vi "CPP_SpectraFit.vi"() -> (5 "Plug in titles":string[](array[string]), 7 "Plug in values":string[](array[string]))   [LabVIEW 2011]
uses:
  Controls/Instrument_Array.ctl
  Controls/Post_Process.ctl
  Controls/Graph_Type.ctl
  Globals/Meas_global.vi
panel:
  in  "Divider":i32(slide)=10 scale=1.0..100000.0 scale format="%#_6e"
  out "dF/ Hz":dbl
  in  "Show Smooth":bool=TRUE
  in  "Save Spectra?":bool
  in  "Desired number of samples per block":i32=32768
  out "Spectra":cluster{"Frequencies":dbl[], dbl[]}[](graph)
  in  "Averaging samples":i32=1 min=1 max=1000
  in  "Spectra Index (from ALL channels)":i32
  out "Waveform Graph":dbl[][](graph)
  in  "Channels to Plot":i32[](array[ring])=[0] items=["RV (Uref)", "Save Nothing"]
  # "Run this VI to update the channel names"
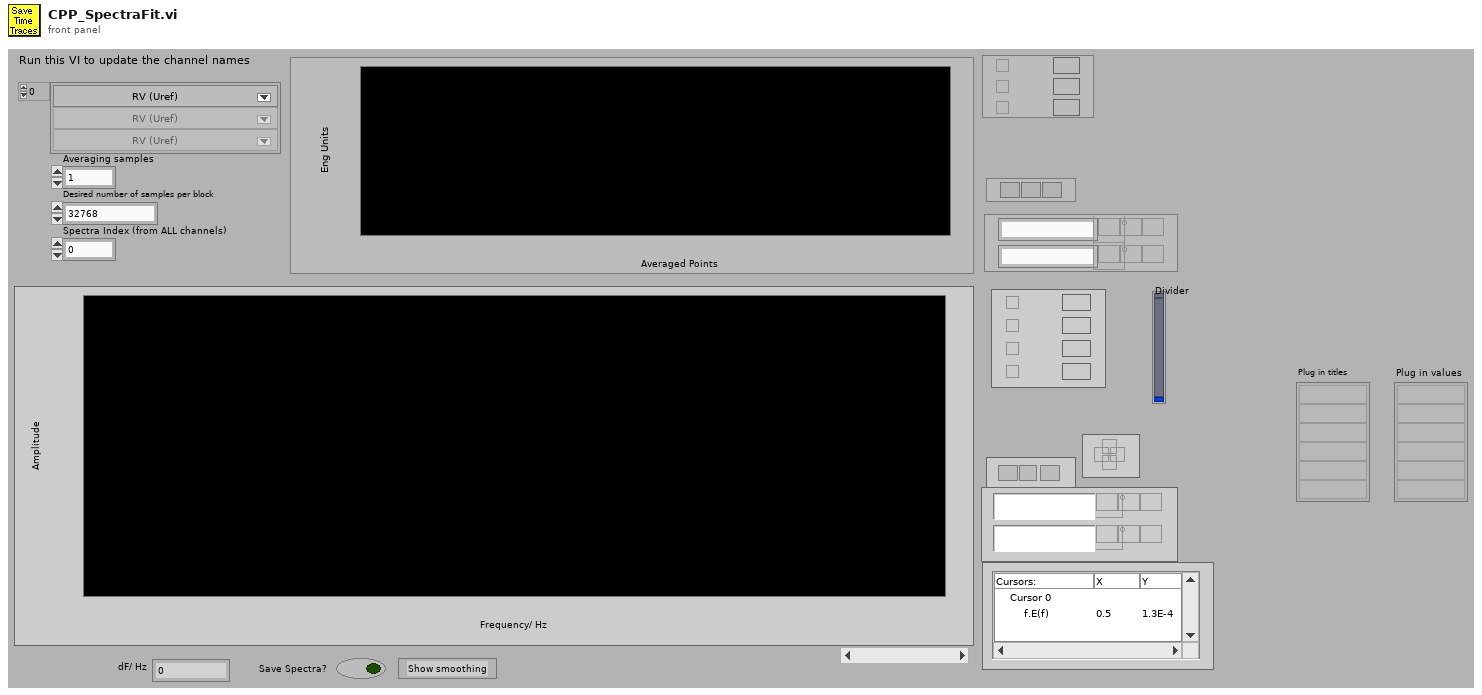
[diagram p1: front panel]
types:
  T1 = typedef "Analysis_info_cluster.ctl" = cluster{"Colour":u32, "Inst type":T2, "Inst name":string, "Symbol":string, "Code name":string, "Extra Info":string, "Inst Array":T3, "Extra Titles":string[], "Extra Values":string[], "U":dbl, "u^2":dbl, "u^3":dbl, "u^4":dbl, "Skew_u":dbl, "Kurt_u":dbl, "Sd Error in Mean":dbl, "% u'/U":dbl, "X":dbl, "Y":dbl, "Z":dbl, "Timescale integral to 25%":dbl, "Sd Error in Variance":dbl, "Calib File":path, "Calib Constants":dbl[], "Output Position":bool, "Full Stats":bool, "Av Sampling Rate":dbl, "Av No of Samples":dbl, "Total Meas Time (s)":dbl, "ADAM Ch Name":string}
  T2 = typedef "Inst_type.ctl" = enum16{"Propeller anemometer", "Raw voltage", "Pressure Transducer", "Pitot-static tube", "Preston tube", "Hot wire", "Cross wire 1", "Cross wire 2", "Generic Linear", "Generic Polynomial", "Generic BackPoly", "Fast FID", "Thermocouple", "Cold wire", "Pulsed Wire", "LDA Vel", "LDA Tran time", "LDA Arr time"}
  T3 = typedef "Instrument_Array.ctl" = enum16{"PWA", "LDA", "Analogue"}
  T4 = typedef "Post_Process.ctl" = enum16{"Take New Data", "Post Process Raw Data File"}
  T5 = typedef "Graph_Type.ctl" = enum16{"Show no graph", "Voltage trace", "Velocity trace", "Vel histogram", "Spectrum", "f.E(f) v Log f", "Auto-Corr"}
  T6 = cluster{"Plot 1":u16, "Plot 2":u16, "Save graph":u16, "Plot Type":T5}
  T7 = cluster{"Weighting":dbl[], "Time (ms)":dbl[], "Voltage":dbl[], "Eng Values":dbl[]}[]
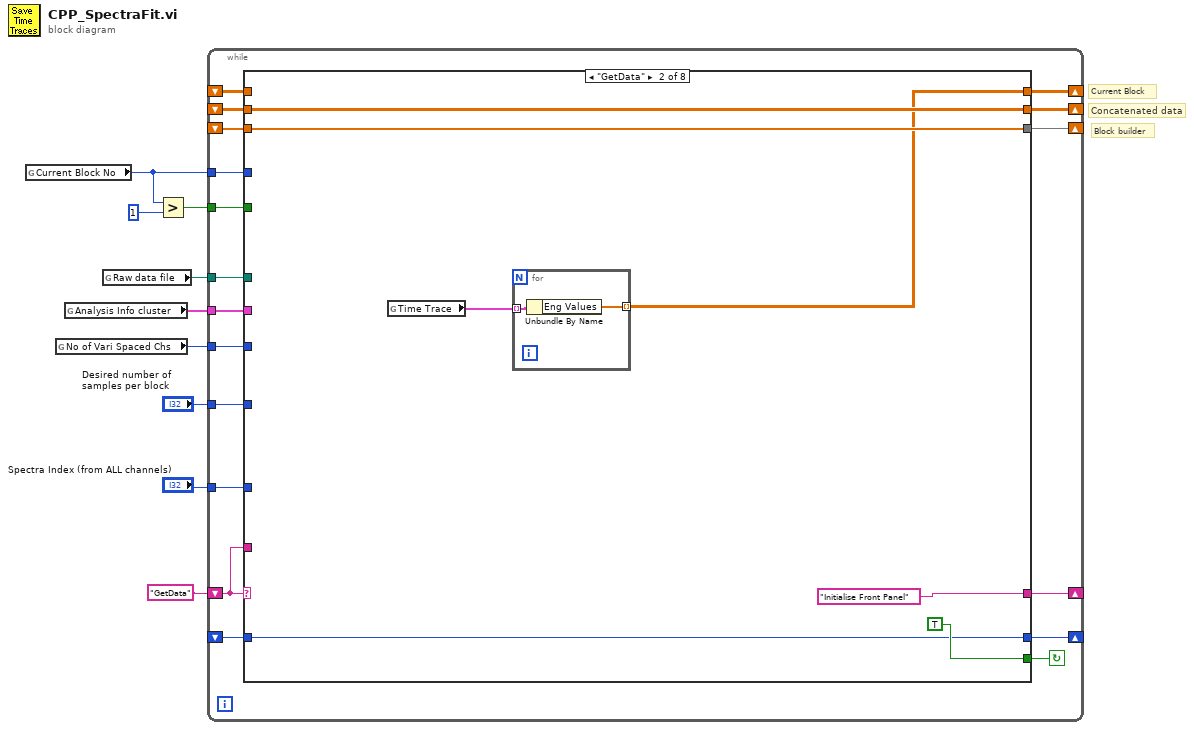
[diagram p0: block diagram]
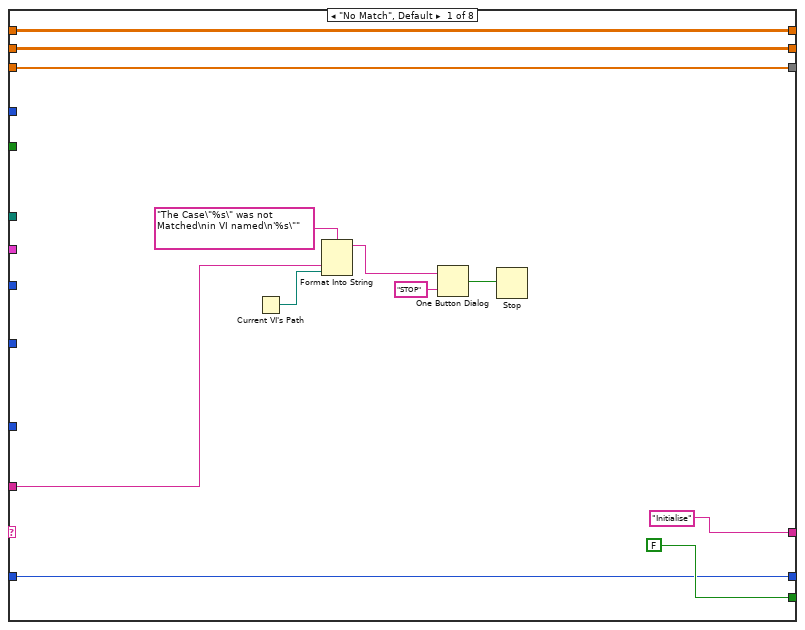
[diagram p2: hidden frame]
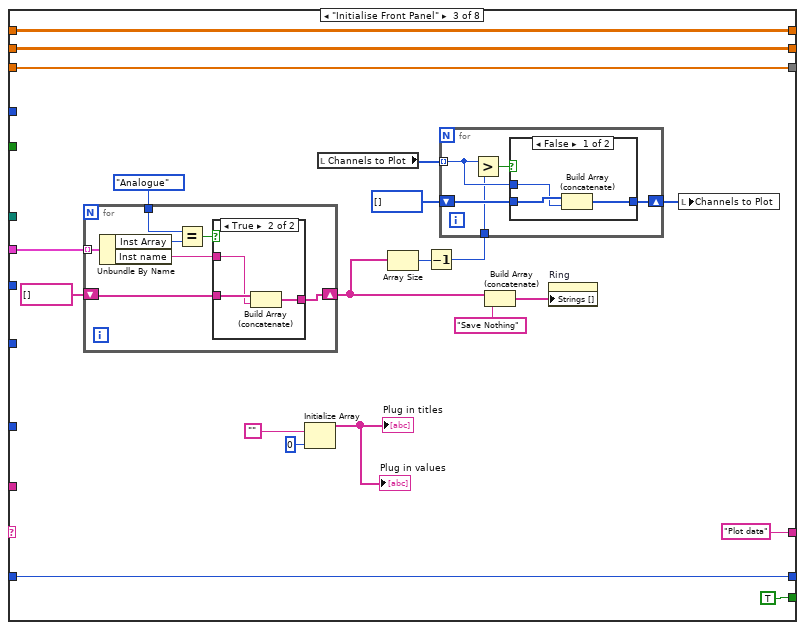
[diagram p3: hidden frame]
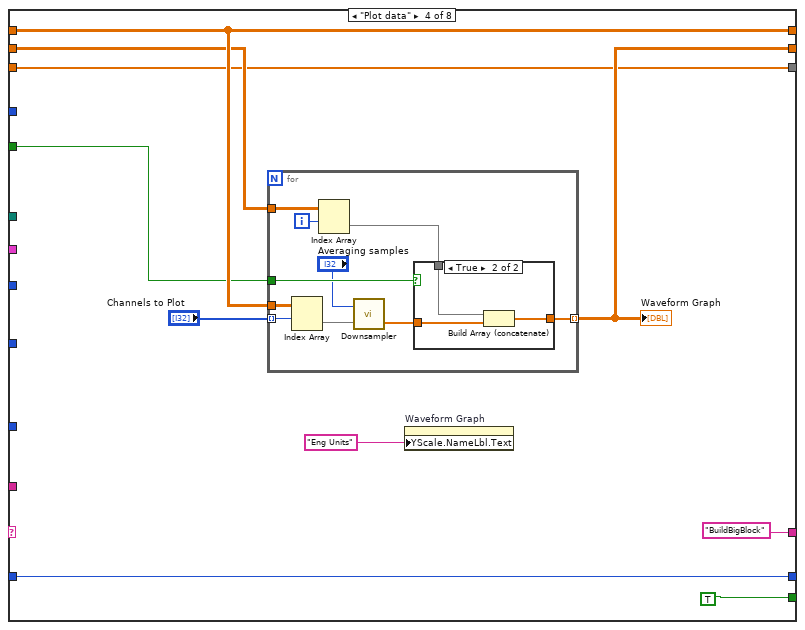
[diagram p6: hidden frame]
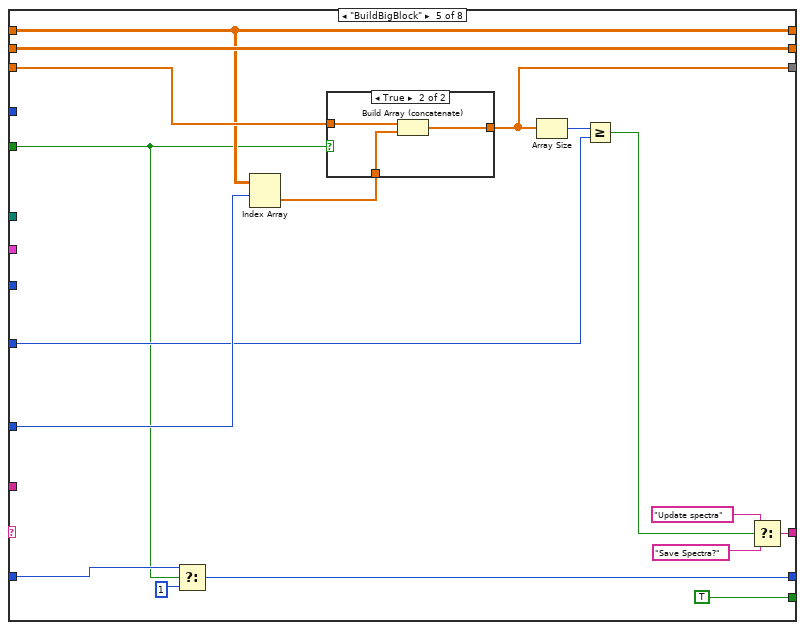
[diagram p8: hidden frame]
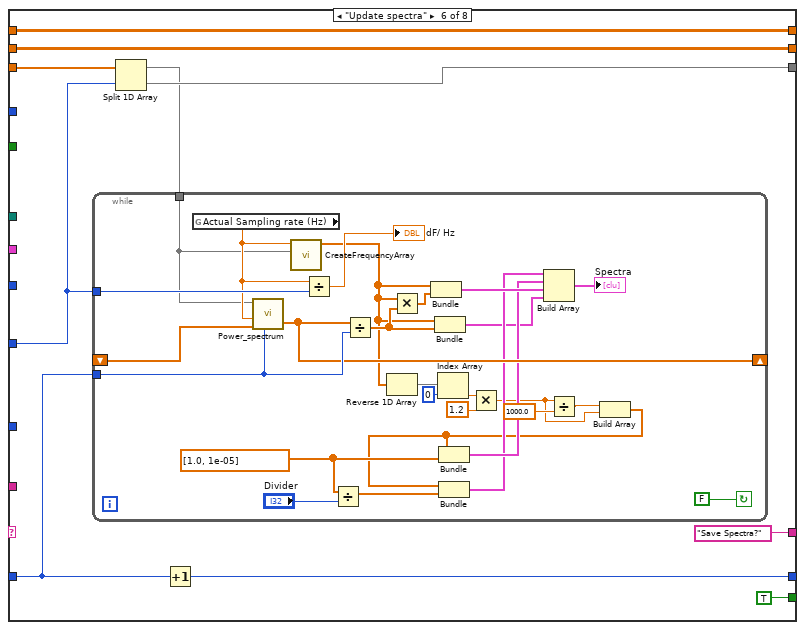
[diagram p10: hidden frame]
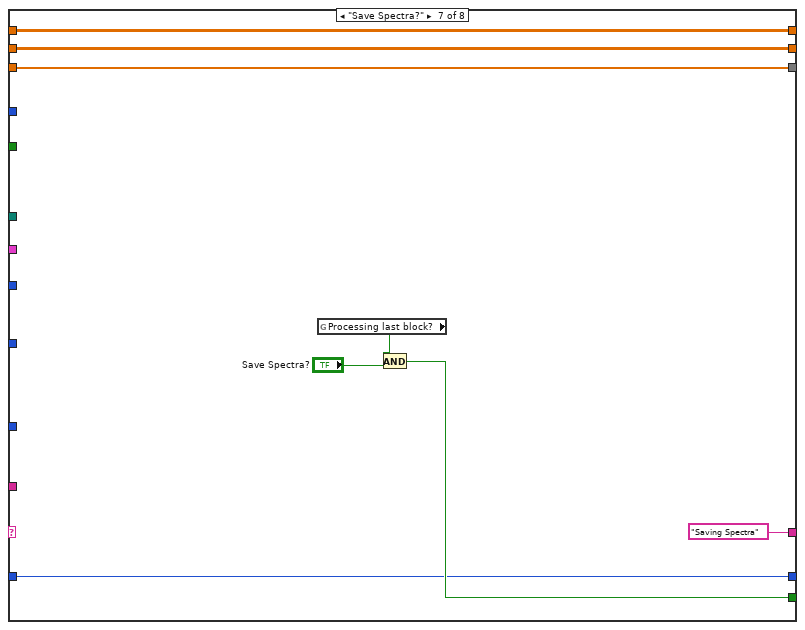
[diagram p11: hidden frame]
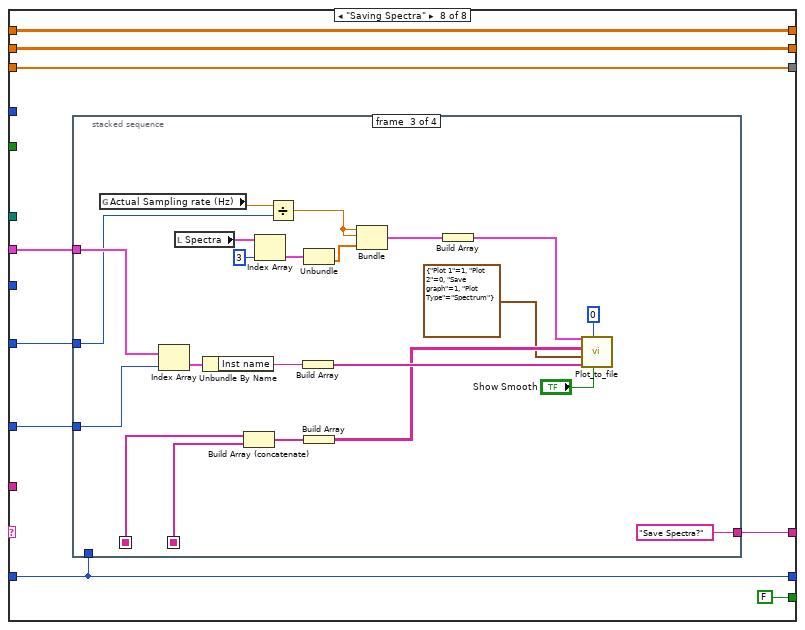
[diagram p12: hidden frame]
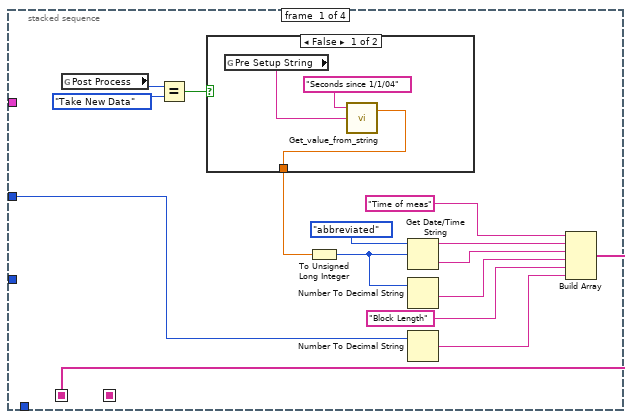
[diagram p13: hidden frame]
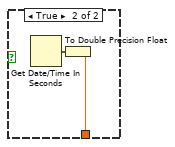
[diagram p14: hidden frame]
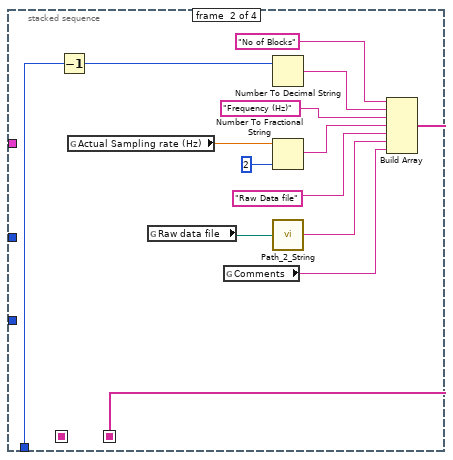
[diagram p15: hidden frame]
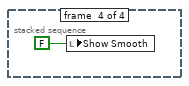
[diagram p16: hidden frame]
diagram:
  # "Block builder"
  # "Concatenated data"
  # "Current Block"
  n1 = global read "Meas_global.vi" "Current Block No"() -> (w6:i32)
  n2 = global read "Meas_global.vi" "No of Vari Spaced Chs"() -> (w4:i32)
  n3 = global read "Meas_global.vi" "Analysis Info cluster"() -> (w5:T1[])
  n4 = global read "Meas_global.vi" "Raw data file"() -> (w8:path)
  n5 = Greater?(x=w6, y=1) -> (0:w3:bool)
  n6 = while {
    shift-left: "GetData" -> [w25]
    shift-right: [w26] -> _
    tunnel: w8 -> [w24]
    tunnel: w3 -> [w23]
    tunnel: w6 -> [w22]
    tunnel: w5 -> [w21]
    tunnel: w4 -> [w20]
    shift-right: [w19] -> _
    shift-left: _ -> [w18]
    shift-right: [w16] -> _
    shift-left: _ -> [w17]
    shift-right: [w14] -> _
    shift-left: _ -> [w15]
    tunnel: "Desired number of samples per block" -> [w13]
    tunnel: "Spectra Index (from ALL channels)" -> [w12]
    shift-right: [w11] -> _
    shift-left: _ -> [w10]
    stop <- w27 continue-if-true
    n7 = case shown="\"GetData\"" w25 {
      tunnel: [FALSE TRUE TRUE TRUE ("Calculate Spectra and Histogram?") TRUE ("Calculate Spectra and Histogram?") TRUE ("Calculate Spectra and Histogram?") w172 FALSE ("Calculate Spectra and Histogram?")] -> w27
      tunnel: ["Initialise" "Initialise Front Panel" "Plot data" "BuildBigBlock" ("t") w114 "Save Spectra?" "Saving Spectra" w185] -> w26
      tunnel: w25 -> [w34 _ _ _ _ _ _ _]
      tunnel: w24 -> [_ _ _ _ _ _ _ _]
      tunnel: w23 -> [_ _ _ w96 w117 _ _ _]
      tunnel: w22 -> [_ _ _ _ _ _ _ _]
      tunnel: w21 -> [_ _ w52 _ _ _ _ w183]
      tunnel: w20 -> [_ _ _ _ _ _ _ _]
      tunnel: [w31 w40 w58 w98 w127 w142 w177 w186] -> w19
      tunnel: w18 -> [w31 _ w58 w98 w127 w142 w177 w186]
      tunnel: w17 -> [w30 w44 w57 w97 w128 w143 w178 w187]
      tunnel: [w30 w44 w57 w94 w128 w143 w178 w187] -> w16
      tunnel: w15 -> [w29 w43 w54 w92 w129 w141 w175 w184]
      tunnel: [w29 w43 w54 w92 w125 w140 w175 w184] -> w14
      tunnel: w13 -> [_ _ _ _ w121 w136 _ w180]
      tunnel: w12 -> [_ _ _ _ w123 _ _ w182]
      tunnel: [w28 w42 w53 w91 w118 w134 w171 w179] -> w11
      tunnel: w10 -> [w28 w42 w53 w91 w119 w135 w171 w179]
      frame "No Match", Default {
        n8 = Current VI's Path() -> (path=w33:path)
        n9 = Format Into String(format string="The Case\"%s\" was not Matched\nin VI named\n'%s\"" ("Format String"), w34, w33) -> (resulting string=w37:string)  [unwired: 2 in, 1 out]
        n10 = One Button Dialog(message=w37, button name ("OK")="STOP") -> (true=w35:bool)
        n11 = Stop(stop? (T)=w35) -> ()
      }
      frame "GetData" {
        n12 = global read "Meas_global.vi" "Time Trace"() -> (w41:T7)
        n13 = for {
          tunnel: w41 -> [w48] mode=indexing
          tunnel: [w47] -> w40 mode=indexing
          n14 = Unbundle By Name(w48) -> ("Eng Values"=w47:dbl[])
        }
      }
      frame "Initialise Front Panel" {
        n15 = for {
          tunnel: Instrument_Array."Analogue" ("Inst Array") -> [w74]
          tunnel: w52 -> [w73] mode=indexing
          shift-right: [w70] -> w51
          shift-left: string[] [] -> [w71]
          n16 = Unbundle By Name(w73) -> ("Inst Array"=w75:T3, "Inst name"=w69:string)
          n17 = Equal?(x=w74, y=w75) -> (x = y?=w72:bool)
          n18 = case shown="True" w72 {
            tunnel: w71 -> [w76 w79]
            tunnel: [w76 w78] -> w70
            tunnel: w69 -> [_ w77]
            frame False {
            }
            frame True {
              n19 = Build Array (concatenate)(w79, w77) -> (w78:string[])
            }
          }
        }
        n20 = Initialize Array("", 0) -> (→"Plug in values" →"Plug in titles":string[])
        n21 = local read "Channels to Plot"() -> (w65:i32[])
        n22 = Array Size(array=w51) -> (size(s)=w60:i32)
        n23 = Decrement(x=w60) -> (x-1=w59:i32)
        n24 = for {
          tunnel: w65 -> [w81] mode=indexing
          shift-right: [w82] -> w63
          shift-left: i32[] [] -> [w83]
          tunnel: w59 -> [w80]
          n25 = Greater?(x=w81, y=w80) -> (0:w84:bool)
          n26 = case shown="False" w84 {
            tunnel: w83 -> [w87 w88]
            tunnel: [w86 w88] -> w82
            tunnel: w81 -> [w85 _]
            frame False {
              n27 = Build Array (concatenate)(w87, w85) -> (w86:i32[])
            }
            frame True {
            }
          }
        }
        n28 = Build Array (concatenate)(w51, "Save Nothing") -> (w61:string[])
        n29 = property on="Ring" class="Ring (strict)"("Strings []"=w61) -> ()  [unwired: 2 in, 2 out]
        n30 = local write "Channels to Plot"(w63) -> ()
      }
      frame "Plot data" {
        n31 = for {
          tunnel: w98 -> [w108]
          tunnel: "Channels to Plot" -> [w107] mode=indexing
          tunnel: w97 -> [w104]
          tunnel: [w105] -> w94 mode=indexing
          tunnel: w96 -> [w106]
          i -> [w103]
          n32 = Index Array(array=w108, index (row)=w107) -> (element=w101:dbl[])  [unwired: 1 in]
          n33 = Index Array(array=w104, index (row)=w103) -> (element=w102:dbl[])  [unwired: 1 in]
          n34 = call "Downsampler.vi"("Input Array"=w101, "Averaging samples"="Averaging samples") -> ("Downsampled Array"=w100:dbl[])  [unwired: 1 out]
          n35 = case shown="True" w106 {
            tunnel: w102 -> [_ w112]
            tunnel: w100 -> [w109 w111]
            tunnel: [w109 w110] -> w105
            frame False {
            }
            frame True {
              n36 = Build Array (concatenate)(w112, w111) -> (w110:dbl[])
            }
          }
        }
        "Waveform Graph" <- w94
        n37 = property on="Waveform Graph" class="WFGraph (strict)"("YScale.NameLbl.Text"="Eng Units") -> ()  [unwired: 2 in, 2 out]
      }
      frame "BuildBigBlock" {
        n38 = Select(t=w119, s=w117, f=1) -> (s? t:f=w118:i32)
        n39 = Index Array(array=w127, index (row)=w123) -> (element=w126:dbl[])  [unwired: 1 in]
        n40 = case shown="True" w117 {
          tunnel: w129 -> [_ w133]
          tunnel: [w130 w132] -> w125
          tunnel: w126 -> [w130 w131]
          frame False {
          }
          frame True {
            n41 = Build Array (concatenate)(w133, w131) -> (w132:dbl[])
          }
        }
        n42 = Array Size(array=w125) -> (size(s)=w124:i32)
        n43 = Greater Or Equal?(x=w124, y=w121) -> (x >= y?=w113:bool)
        n44 = Select(t="Update spectra", s=w113, f="Save Spectra?") -> (s? t:f=w114:string)
      }
      frame "Update spectra" {
        n45 = Split 1D Array(array=w141, index=w136) -> (first subarray=w137:dbl[], second subarray=w140:dbl[])
        n46 = while {
          shift-left: _ -> [w165]
          shift-right: [w166] -> _
          tunnel: w137 -> [w163]
          tunnel: w135 -> [w169]
          tunnel: w136 -> [w168]
          stop <- FALSE continue-if-true
          w158 = dbl[] [1.0, 1e-05]
          n47 = global read "Meas_global.vi" "Actual Sampling rate (Hz)"() -> (w164:dbl)
          n48 = call "Power_spectrum.vi"("U"=w163, "Sampling frequency"=w164, "Spectrum input array"=w165, "Block No"=w169) -> ("Spectrum output array"=w166:dbl[])  [unwired: 1 in, 1 out]
          n49 = call "CreateFrequencyArray.vi"("Signal"=w163, "Actual Sampling rate (Hz)"=w164) -> ("Frequencies"=w152:dbl[])  [unwired: 9 in]
          n50 = Divide(x=w164, y=w168) -> (x/y=→"dF/ Hz":dbl)
          n51 = Divide(x=w158, y="Divider") -> (x/y=w159:dbl[])
          n52 = Divide(x=w166, y=w169) -> (x/y=w154:dbl[])
          n53 = Reverse 1D Array(array=w152) -> (reversed array=w151:dbl[])
          n54 = Multiply(x=w152, y=w154) -> (x*y=w155:dbl[])
          n55 = Bundle("Frequencies"=w152, w155) -> (w161:cluster{"Frequencies":dbl[], dbl[]})  [unwired: 1 in]
          n56 = Bundle("Frequencies"=w152, w154) -> (w153:cluster{"Frequencies":dbl[], dbl[]})  [unwired: 1 in]
          n57 = Index Array(array=w151, index=0) -> (element=w149:dbl)
          n58 = Multiply(x=w149, y=1.2) -> (x*y=w145:dbl)
          n59 = Divide(x=w145, y=1000.0) -> (x/y=w146:dbl)
          n60 = Build Array(w146, w145) -> (w144:dbl[])
          n61 = Bundle(w144, w158) -> (w160:cluster{dbl[], dbl[]})  [unwired: 1 in]
          n62 = Bundle(w144, w159) -> (w156:cluster{dbl[], dbl[]})  [unwired: 1 in]
          n63 = Build Array(w156, w160, w161, w153) -> (→"Spectra":cluster{"Frequencies":dbl[], dbl[]}[])
        }
        n64 = Increment(x=w135) -> (x+1=w134:i32)
      }
      frame "Save Spectra?" {
        n65 = global read "Meas_global.vi" "Processing last block?"() -> (w173:bool)
        n66 = And(x=w173, y="Save Spectra?") -> (x .and. y?=w172:bool)
      }
      frame "Saving Spectra" {
        n67 = stacked-sequence {
          seq-local: [w191 _ _ _] -> [_ _ w233 _]
          seq-local: [_ w211 _ _] -> [_ _ w232 _]
          tunnel: [_ _ "Save Spectra?" _] -> w185
          tunnel: w183 -> [_ _ w239 _]
          tunnel: w182 -> [_ _ w238 _]
          tunnel: w180 -> [w189 _ w224 _]
          tunnel: w179 -> [_ w209 _ _]
          frame #0 {
            n68 = global read "Meas_global.vi" "Post Process"() -> (w193:T4)
            n69 = Equal?(x=w193, y=Post_Process."Take New Data" ("Post Process")) -> (x = y?=w194:bool)
            n70 = case shown="False" w194 {
              tunnel: [w202 w206] -> w195
              frame False {
                n71 = global read "Meas_global.vi" "Pre Setup String"() -> (w203:string)
                n72 = call "Get_value_from_string.vi"("Input string"=w203, "Variable name"="Seconds since 1/1/04") -> ("Value"=w202:dbl)  [unwired: 1 in, 1 out]
              }
              frame True {
                n73 = Get Date/Time In Seconds() -> (seconds since 1Jan1904=w205:timestamp)
                n74 = To Double Precision Float(number=w205) -> (double precision float=w206:dbl)
              }
            }
            n75 = To Unsigned Long Integer(number=w195) -> (unsigned 32bit integer=w199:u32)
            n76 = Get Date/Time String(date format (0)=enum16{"short", "long", "abbreviated"}."abbreviated", seconds (now)=w199) -> (date string=w197:string, time string=w198:string)  [unwired: 1 out]
            n77 = Number To Decimal String(number=w199) -> (decimal integer string=w200:string)  [unwired: 1 out]
            n78 = Number To Decimal String(number=w189) -> (decimal integer string=w188:string)  [unwired: 1 out]
            n79 = Build Array("Time of meas", w197, w198, w200, "Block Length" ("element"), w188) -> (w191:string[])
          }
          frame #1 {
            n80 = Decrement(x=w209) -> (x-1=w208:i32)
            n81 = global read "Meas_global.vi" "Actual Sampling rate (Hz)"() -> (w212:dbl)
            n82 = global read "Meas_global.vi" "Raw data file"() -> (w218:path)
            n83 = global read "Meas_global.vi" "Comments"() -> (w217:string)
            n84 = Number To Decimal String(number=w208) -> (decimal integer string=w207:string)  [unwired: 1 out]
            n85 = Number To Fractional String(number=w212, precision (6)=i16 2) -> (F-format string=w215:string)  [unwired: 2 out]
            n86 = call "Path_2_String.vi"("Real Path"=w218) -> ("Path String"=w219:string)
            n87 = Build Array("No of Blocks", w207, "Frequency (Hz)", w215, "Raw Data file", w219, w217) -> (w211:string[])
          }
          frame #2 {
            n88 = global read "Meas_global.vi" "Actual Sampling rate (Hz)"() -> (w225:dbl)
            n89 = Index Array(array=w239, index=w238) -> (element=w237:T1)
            n90 = local read "Spectra"() -> (w228:cluster{"Frequencies":dbl[], dbl[]}[])
            n91 = Unbundle By Name(w237) -> ("Inst name"=w236:string)
            n92 = Build Array (concatenate)(w233, w232) -> (w231:string[])
            n93 = Index Array(array=w228, index=3) -> (element=w226:cluster{"Frequencies":dbl[], dbl[]})
            n94 = Divide(x=w225, y=w224) -> (x/y=w222:dbl)
            n95 = Build Array(w236) -> (w235:string[])
            n96 = Unbundle(w226) -> (w223:dbl[])  [unwired: 1 out]
            n97 = Build Array(w231) -> (w230:string[][])
            n98 = Bundle(w222, w222, w223) -> (w221:cluster{dbl, dbl, dbl[]})  [unwired: 1 in]
            n99 = Build Array(w221) -> (w220:cluster{dbl, dbl, dbl[]}[])
            n100 = call "Plot_to_file.vi"("Show Smooth"="Show Smooth", "Start trace No"=0, "Trace names"=w235, "Graph"=T6 {"Plot 1"=1, "Plot 2"=0, "Save graph"=1, "Plot Type"=enum."Spectrum"}, "Plot file label"=w230, "Plot data"=w220) -> ()  [unwired: 6 out]
          }
          frame #3 {
            n101 = local write "Show Smooth"(FALSE ("Show Smooth")) -> ()
          }
        }
      }
    }
  }
